vi "Content.vi"(7 "Context":refnum<class "Context.lvclass">, 8 "Error In":errorcluster, 11 "Template In":refnum<class "Root.lvclass">) -> (0 "Error Out":errorcluster, 2 "Content":string, 3 "Template Out":refnum<class "Root.lvclass">)   [LabVIEW 2018, in "Toolkit.lvlib" / "Nodes.lvlib" / "Root.lvclass"]
uses:
  Root.lvclass
  Support/Context/Context.lvclass
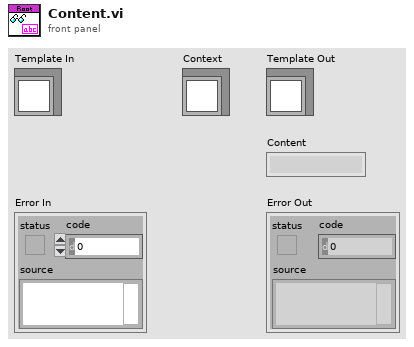
[diagram p1: front panel]
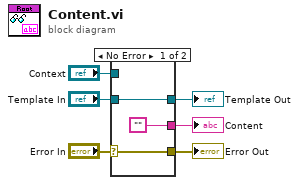
[diagram p0: block diagram]
diagram:
  n1 = case shown="No Error" "Error In" {
    selector: "Error In" -> [w9 w11]
    tunnel: [w9 w11] -> w5
    tunnel: "Template In" -> [w8 w10]
    tunnel: [w8 w10] -> w3
    tunnel: ["" _] -> w2
    tunnel: "Context" -> [_ _]
    frame No Error {
    }
    frame Error {
    }
  }
  "Error Out" <- w5
  "Template Out" <- w3
  "Content" <- w2
